vi "populate kvp table.vi"(8 "error in":errorcluster, 10 "MCListbox Refnum":refnum<vi>, 11 "fixed channel configuration in":refnum<class "fixed channel configuration.lvclass">) -> (0 "error out":errorcluster)   [LabVIEW 2013, in "fixed channel editor.lvclass"]
uses:
  fixed channel editor.lvclass
  module/configuration/fixed channel configuration.lvclass
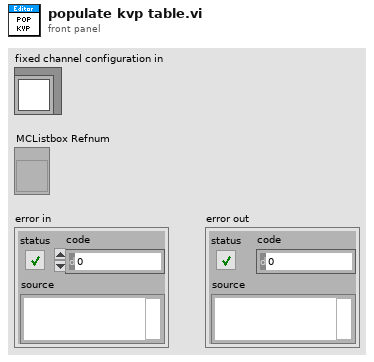
[diagram p1: front panel]
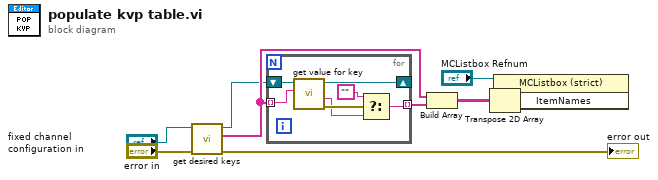
[diagram p0: block diagram]
diagram:
  n1 = call-dynamic "get desired keys.vi"("error in"="error in", "fixed channel configuration in"="fixed channel configuration in") -> ("error out"=→"error out":errorcluster, "desired keys"=w8:string[], "fixed channel configuration out"=w5:refnum<class "fixed channel configuration.lvclass">)  [unwired: 7 in]
  n2 = for {
    shift-right: [w15] -> _
    shift-left: w5 -> [w16]
    tunnel: w8 -> [w14] mode=indexing
    tunnel: [w10] -> w6 mode=indexing
    n3 = call-dynamic "get value for key.vi"("key"=w14, "fixed channel configuration in"=w16) -> ("error out"=w13:errorcluster, "value"=w12:string, "fixed channel configuration out"=w15:refnum<class "fixed channel configuration.lvclass">)  [unwired: 7 in]
    n4 = Select(t="", s=w13, f=w12) -> (s? t:f=w10:string)
  }
  n5 = Build Array(w8, w6) -> (w7:string[][])
  n6 = Transpose 2D Array(2D array=w7) -> (transposed array=w9:string[][])
  n7 = property on="Property Node" class="MCListbox (strict)"(reference="MCListbox Refnum", "ItemNames"=w9) -> ()  [unwired: 1 in, 2 out]
